vi "IMUOrientClose.vi"(11 "IMU Dev Ref":T1={"I2CDevRef"={"DevStatus"={"status"=FALSE, "code"=0, "source"=""}, "Device Address"=0, "Handle"=0, "I2C Bus"=enum."Invalid"}, "Valid Cal File?"=FALSE} {"I2CDevRef"."Device Address" format="%.0x"}) -> ()   [LabVIEW 2017]
uses:
  <userlib>/836-Library/Sensor/IMU/ImuDevRef.ctl
  <vilib>/Rock Robotics/WPI/I2C/WPI_I2CDevRef.ctl
  <vilib>/Rock Robotics/SystemInterfaces/i2clib/i2c_bus.ctl
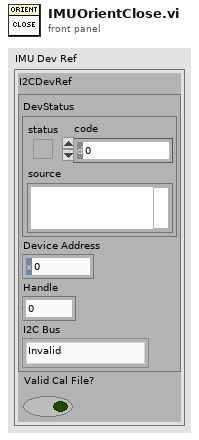
[diagram p1: front panel]
types:
  T1 = typedef "ImuDevRef.ctl" = cluster{"I2CDevRef":T2, "Valid Cal File?":bool}
  T2 = typedef "WPI_I2CDevRef.ctl" = cluster{"DevStatus":errorcluster, "Device Address":u8, "Handle":i32, "I2C Bus":T3}
  T3 = typedef "i2c_bus.ctl" = enum16{"I2C On-Board", "I2C MXP", "Invalid"}
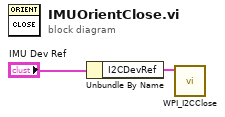
[diagram p0: block diagram]
diagram:
  n1 = Unbundle By Name("IMU Dev Ref") -> ("I2CDevRef"=w1:T2)
  n2 = call <vilib>:"WPI_I2CClose.vi"("I2CDevRef"=w1) -> ()  [unwired: 10 in, 1 out]
